vi "Get Python Path.vi"(8 "error in (no error)":errorcluster, 10 "Python Rev Key":string) -> (0 "error out":errorcluster, 3 "Python.exe path":string)   [LabVIEW 2022 SP3]
doc: "Get Python Path output Python.exe path\nIt allows entering Python rev keyword to select specific rev that installed on the computer"
uses:
  <vilib>/Utility/error.llb/Trim Whitespace One-Sided.vi
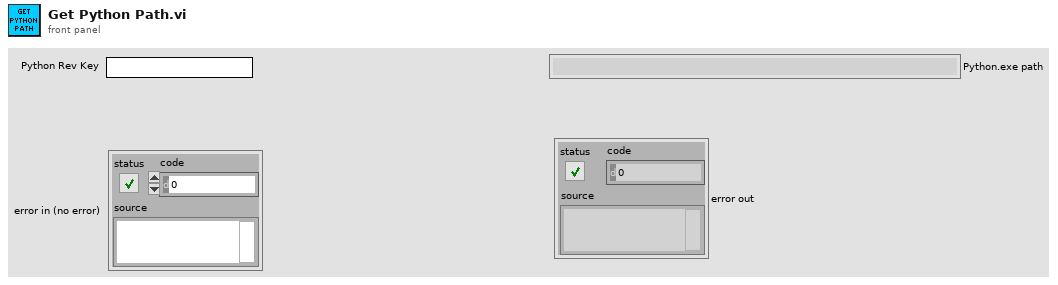
[diagram p1: front panel]
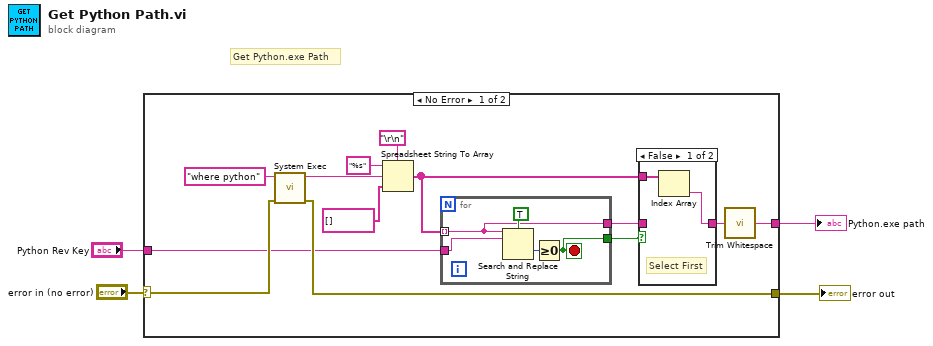
[diagram p0: block diagram]
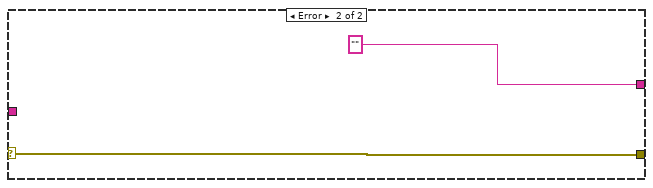
[diagram p3: hidden frame]
diagram:
  # "Get Python.exe Path"
  n1 = case shown="No Error" "error in (no error)" {
    selector: "error in (no error)" -> [w10 w27]
    tunnel: [w12 "" ("trimmed string")] -> w4
    tunnel: [w11 w27] -> w3
    tunnel: "Python Rev Key" -> [w9 _]
    frame No Error {
      n2 = call <vilib>:"System Exec.vi"("error in (no error)"=w10, "command line"="where python") -> ("error out"=w11:errorcluster, "standard output"=w17:string)  [unwired: 6 in, 2 out]
      n3 = Spreadsheet String To Array(delimiter (Tab)="\r\n", format string="%s", spreadsheet string=w17, array type (2D Dbl)=string[] []) -> (array=w7:string[])
      n4 = for {
        tunnel: w7 -> [w22] mode=indexing
        tunnel: w9 -> [w25]
        tunnel: [w22] -> w6
        tunnel: [w21] -> w8
        stop <- w21 stop-if-true
        n5 = Search and Replace String(case sensitive?=TRUE ("ignore case? (F)"), input string=w22, search string=w25) -> (offset past replacement=w23:i32)  [unwired: 5 in, 3 out]
        n6 = Greater Or Equal To 0?(x=w23) -> (x >= 0?=w21:bool)
      }
      n7 = case shown="False" w8 {
        tunnel: w7 -> [w19 _]
        tunnel: w6 -> [_ w20]
        tunnel: [w18 w20] -> w5
        frame False {
          # "Select First"
          n8 = Index Array(array=w19) -> (element=w18:string)  [unwired: 1 in]
        }
        frame True {
          # "Found Key"
        }
      }
      n9 = call <vilib>:"Trim Whitespace.vi"("string"=w5) -> ("trimmed string"=w12:string)  [unwired: 1 in]
    }
    frame Error {
    }
  }
  "Python.exe path" <- w4
  "error out" <- w3
